vi "Data_To_String_Array.vi"(5 "MODE":string, 7 "TSN":string, 8 "Hardness_string":string[](array[string]), 9 "DIN":string, 10 "Test_load_string":string[](array[string]), 11 "TEMP":string) -> (2 "String_Array":string[][](array[string]))   [LabVIEW 2019]
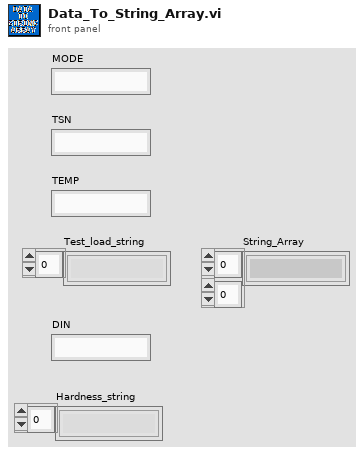
[diagram p1: front panel]
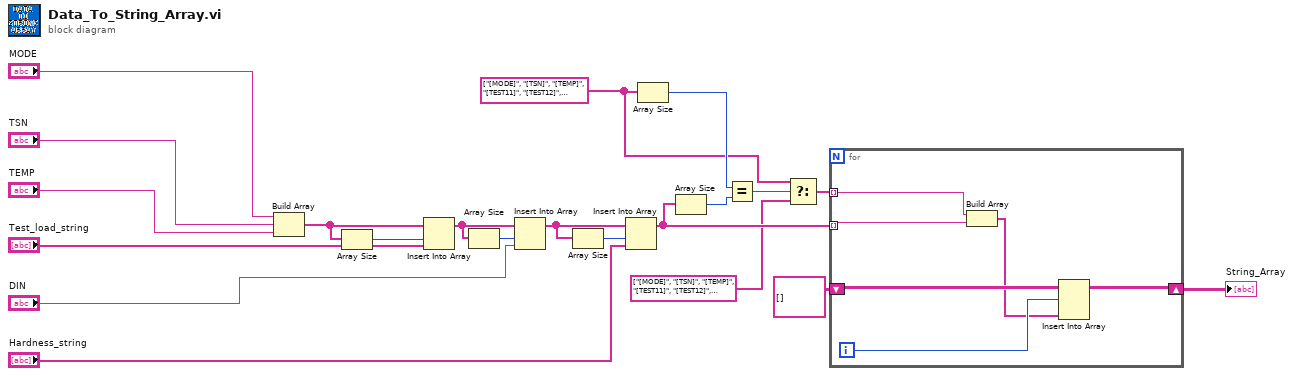
[diagram p0: block diagram]
diagram:
  w1 = string[] ["[MODE]", "[TSN]", "[TEMP]", "[TEST11]", "[TEST12]", "[TEST13]", "[DEV1]", "[INACC1]", "[TEST21]", "[TEST22]", "[TEST23]", "[DEV2]", "[INACC2]", "[TEST31]", "[TEST32]", "[TEST33]", "[DEV3]", "[INACC3]", "[TEST41]", "[TEST42]", "[TEST43]", "[DEV4]", "[INACC4]", "[DIN]", "[HN1]", "[HS1]", "[TV11]", "[TV12]", "[TV13]", "[TV14]", "[TV15]", "[AVG1]", "[HV1]", "[REP1]", "[HN2]", "[HS2]", "[TV21]", "[TV22]", "[TV23]", "[TV24]", "[TV25]", "[AVG2]", "[HV2]", "[REP2]", "[HN3]", "[HS3]", "[TV31]", "[TV32]", "[TV33]", "[TV34]", "[TV35]", "[AVG3]", "[HV3]", "[REP3]", "[HN4]", "[HS4]", "[TV41]", "[TV42]", "[TV43]", "[TV44]", "[TV45]", "[AVG4]", "[HV4]", "[REP4]", "[HN5]", "[HS5]", "[TV51]", "[TV52]", "[TV53]", "[TV54]", "[TV55]", "[AVG5]", "[HV5]", "[REP5]"] ("待写入项")
  n1 = Build Array("MODE", "TSN", "TEMP") -> (w11:string[])
  n2 = Array Size(array=w11) -> (size(s)=w12:i32)
  n3 = Insert Into Array(array=w11, index=w12, new element="Test_load_string") -> (w15:string[])
  n4 = Array Size(array=w15) -> (size(s)=w14:i32)
  n5 = Insert Into Array(array=w15, index=w14, new element="DIN") -> (w17:string[])
  n6 = Array Size(array=w17) -> (size(s)=w18:i32)
  n7 = Insert Into Array(array=w17, index=w18, new element="Hardness_string") -> (w7:string[])
  n8 = Array Size(array=w1) -> (size(s)=w3:i32)
  n9 = Array Size(array=w7) -> (size(s)=w6:i32)
  n10 = Equal?(x=w3, y=w6) -> (x = y?=w4:bool)
  n11 = Select(t=w1, s=w4, f=string[] ["[MODE]", "[TSN]", "[TEMP]", "[TEST11]", "[TEST12]", "[TEST13]", "[DEV1]", "[INACC1]", "[TEST21]", "[TEST22]", "[TEST23]", "[DEV2]", "[INACC2]", "[TEST31]", "[TEST32]", "[TEST33]", "[DEV3]", "[INACC3]", "[TEST41]", "[TEST42]", "[TEST43]", "[DEV4]", "[INACC4]", "[TEST51]", "[TEST52]", "[TEST53]", "[DEV5]", "[INACC5]", "[TEST61]", "[TEST62]", "[TEST63]", "[DEV6]", "[INACC6]", "[TEST71]", "[TEST72]", "[TEST73]", "[DEV7]", "[INACC7]", "[TEST81]", "[TEST82]", "[TEST83]", "[DEV8]", "[INACC8]", "[DIN]", "[HN1]", "[HS1]", "[TV11]", "[TV12]", "[TV13]", "[TV14]", "[TV15]", "[AVG1]", "[HV1]", "[REP1]", "[HN2]", "[HS2]", "[TV21]", "[TV22]", "[TV23]", "[TV24]", "[TV25]", "[AVG2]", "[HV2]", "[REP2]", "[HN3]", "[HS3]", "[TV31]", "[TV32]", "[TV33]", "[TV34]", "[TV35]", "[AVG3]", "[HV3]", "[REP3]", "[HN4]", "[HS4]", "[TV41]", "[TV42]", "[TV43]", "[TV44]", "[TV45]", "[AVG4]", "[HV4]", "[REP4]", "[HN5]", "[HS5]", "[TV51]", "[TV52]", "[TV53]", "[TV54]", "[TV55]", "[AVG5]", "[HV5]", "[REP5]"] ("待写入项")) -> (s? t:f=w5:string[])
  n12 = for {
    tunnel: w5 -> [w22] mode=indexing
    tunnel: w7 -> [w27] mode=indexing
    shift-right: [w24] -> w21
    shift-left: string[][] [] -> [w26]
    i -> [w25]
    n13 = Build Array(w22, w27) -> (w23:string[])
    n14 = Insert Into Array(array=w26, index (row)=w25, new element=w23) -> (w24:string[][])  [unwired: 1 in]
  }
  "String_Array" <- w21
